vi "TalonSRXConfigPID.vi"(0 "Device Reference (in)":T1, 1 "PID Slot":i32, 5 "PID Parameters":T6, 11 "Error (in)":errorcluster) -> (4 "Device Reference (out)":T1, 15 "Error (out)":errorcluster)   [LabVIEW 2020]
doc: "Wrapper for configuring the PID on a Talon SRX motor controller."
uses:
  5ec5a0a5-e256-4685-9647-f7ac00e8f22e.vi
  <vilib>/Rock Robotics/SystemInterfaces/DIO/FPGA_DIOPWMChannel.ctl
  <vilib>/Rock Robotics/WPI/PWM/WPI_PWMDeadband.ctl
  <vilib>/Rock Robotics/WPI/MotorControl/WPI_MotorControlType.ctl
  <vilib>/Rock Robotics/SystemInterfaces/DIO/FPGA_DIOChannel.ctl
  <vilib>/Rock Robotics/WPI/MotorControl/WPI_MotorControlDeviceRef.ctl
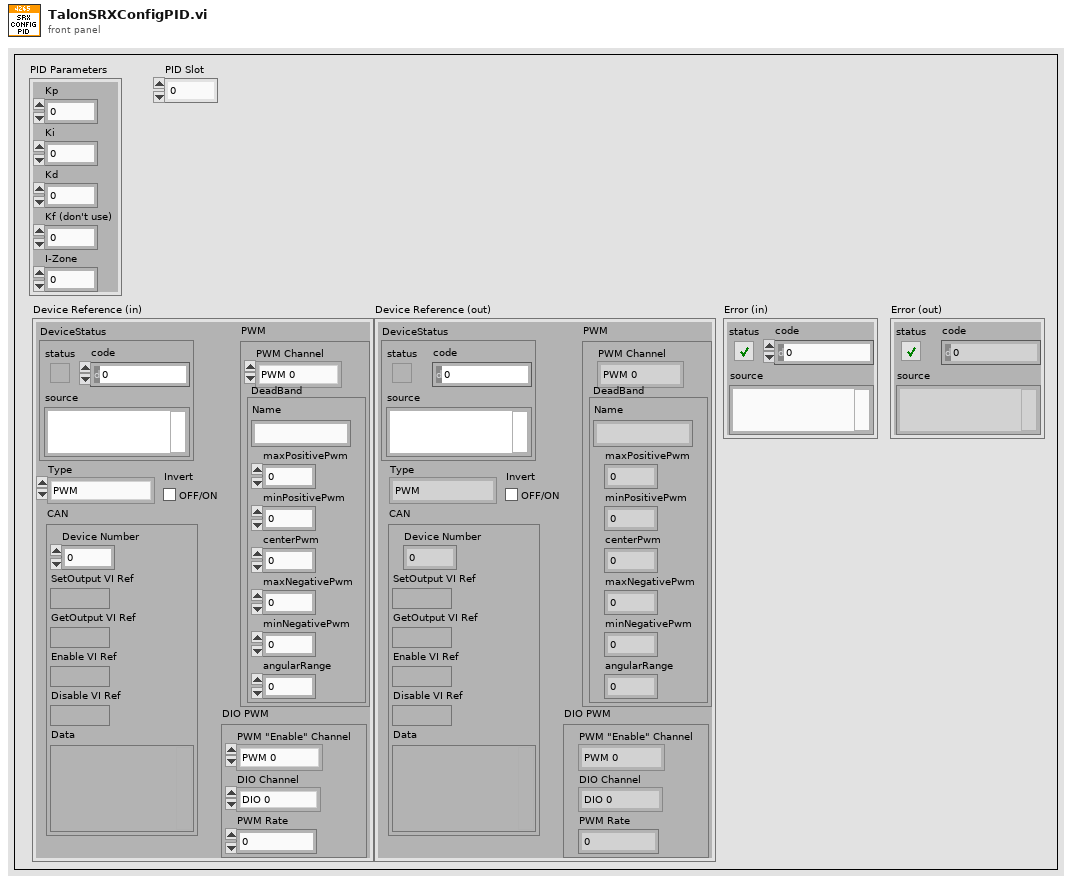
[diagram p1: front panel]
types:
  T1 = typedef "WPI_MotorControlDeviceRef.ctl" = cluster{"DeviceStatus":errorcluster, "Type":T2, "PWM":cluster{"PWM Channel":T3, "DeadBand":T4}, "CAN":cluster{"Device Number":u8, "SetOutput VI Ref":variant, "GetOutput VI Ref":variant, "Enable VI Ref":variant, "Disable VI Ref":variant, "Data":variant}, "Invert":bool, "DIO PWM":cluster{"PWM \"Enable\" Channel":T3, "DIOChannel":T5, "PWM Rate":dbl}}
  T2 = typedef "WPI_MotorControlType.ctl" = enum16{"PWM", "CAN", "DIO PWM"}
  T3 = typedef "FPGA_DIOPWMChannel.ctl" = enum8{"PWM 0", "PWM 1", "PWM 2", "PWM 3", "PWM 4", "PWM 5", "PWM 6", "PWM 7", "PWM 8", "PWM 9", "PWM MXP 0", "PWM MXP 1", "PWM MXP 2", "PWM MXP 3", "PWM MXP 4", "PWM MXP 5", "PWM MXP 6", "PWM MXP 7", "PWM MXP 8", "PWM MXP 9", "Invalid"}
  T4 = typedef "WPI_PWMDeadband.ctl" = cluster{"Name":string, "maxPositivePwm":i32, "minPositivePwm":i32, "centerPwm":i32, "maxNegativePwm":i32, "minNegativePwm":i32, "angularRange":u16}
  T5 = typedef "FPGA_DIOChannel.ctl" = enum8{"DIO 0", "DIO 1", "DIO 2", "DIO 3", "DIO 4", "DIO 5", "DIO 6", "DIO 7", "DIO 8", "DIO 9", "DIO MXP 0", "DIO MXP 1", "DIO MXP 2", "DIO MXP 3", "DIO MXP 4", "DIO MXP 5", "DIO MXP 6", "DIO MXP 7", "DIO MXP 8", "DIO MXP 9", "DIO MXP 10", "DIO MXP 11", "DIO MXP 12", "DIO MXP 13", "DIO MXP 14", "DIO MXP 15", "SPI Port CS1", "SPI Port CS2", "SPI Port CS3", "SPI Port MISO", "SPI Port MOSI", "Invalid"}
  T6 = cluster{"Kp":dbl, "Ki":dbl, "Kd":dbl, "Kf (don't use)":dbl, "I-Zone":dbl}
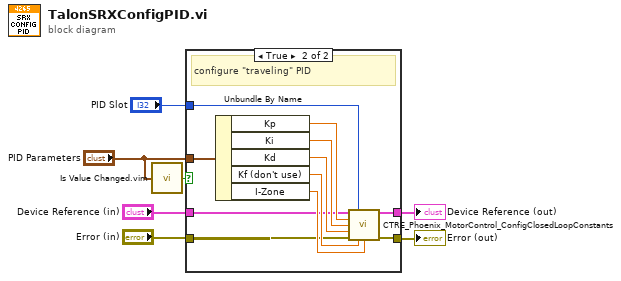
[diagram p0: block diagram]
diagram:
  n1 = call "Is Value Changed.vim"("value"="PID Parameters") -> ("changed or first call?"=w3:bool)
  n2 = case shown="True" w3 {
    tunnel: "PID Parameters" -> [_ w17]
    tunnel: "Device Reference (in)" -> [w9 w14]
    tunnel: "Error (in)" -> [w8 w13]
    tunnel: [w9 w12] -> w5
    tunnel: [w8 w11] -> w6
    tunnel: "PID Slot" -> [_ w10]
    frame False {
    }
    frame True {
      # "configure \"traveling\" PID"
      n3 = Unbundle By Name(w17) -> ("Kp"=w18:dbl, "Ki"=w19:dbl, "Kd"=w20:dbl, "Kf (don't use)"=w16:dbl, "I-Zone"=w15:dbl)
      n4 = call <vilib>:"CTRE_Phoenix_MotorControl_ConfigClosedLoopConstants.vi"("PhoenixMotorControlDevRef"=w14, "slotIdx"=w10, "P"=w18, "I"=w19, "D"=w20, "error in (no error)"=w13, "F"=w16, "I Zone"=w15) -> ("PhoenixMotorControlDevRef"=w12:T1, "error out"=w11:errorcluster)  [unwired: 6 in]
    }
  }
  "Error (out)" <- w6
  "Device Reference (out)" <- w5
